vi "IsWatingForUpdate.vi"(8 "error in (no error)":errorcluster, 11 "BME_DG_System in":refnum<class "BME_DG_System.lvclass">) -> (0 "error out":errorcluster, 2 "StillWaiting":bool, 3 "BME_DG_System out":refnum<class "BME_DG_System.lvclass">)   [LabVIEW 2009, in "POLARIS BME DG.lvlib" / "BME_DG_System.lvclass"]
uses:
  BME_DG_System.lvclass
  POLARIS BME DG.lvlib
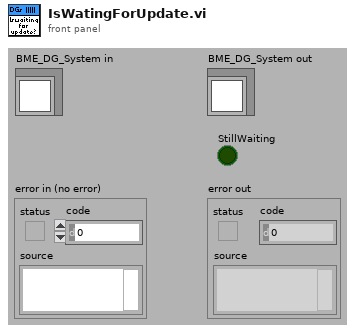
[diagram p1: front panel]
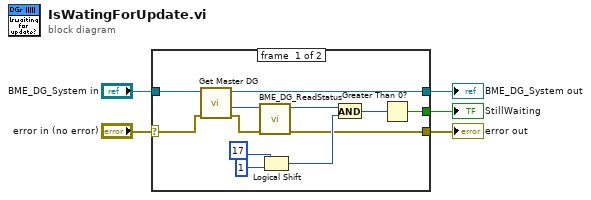
[diagram p0: block diagram]
diagram:
  n1 = case shown="No Error" "error in (no error)" {
    selector: "error in (no error)" -> [w15 w19]
    tunnel: [w7 w19] -> w4
    tunnel: [w16 w18] -> w2
    tunnel: "BME_DG_System in" -> [w17 w18]
    tunnel: [w6 _] -> w1
    frame #0 {
      n2 = call "Get Master DG.vi"("error in (no error)"=w15, "BME_DG_System in"=w17) -> ("error out"=w13:errorcluster, "MasterDGNr"=w14:i32, "BME_DG_System out"=w16:refnum<class "BME_DG_System.lvclass">)  [unwired: 6 in, 1 out]
      n3 = call "BME_DG_ReadStatus.vi"("error in (no error)"=w13, "DG_Number"=w14) -> ("error out"=w7:errorcluster, "return value"=w10:i32)  [unwired: 8 in]
      n4 = Logical Shift(y=i8 17, x=u32 1) -> (x << y=w9:u32)
      n5 = And(x=w10, y=w9) -> (x .and. y?=w8:u32)
      n6 = Greater Than 0?(x=w8) -> (x > 0?=w6:bool)
    }
    frame #1 {
    }
  }
  "error out" <- w4
  "BME_DG_System out" <- w2
  "StillWaiting" <- w1
